vi "BLM Control Text In.vi"(1 "command text in":string[](array[string])=["N/A", "Magent PS", "N/A", "Set Field", "Set Field to 2.0000E+0 @ 0.0000T /min, no wait , extra 0 sec wait", "N/A", "N/A", "", "1", "0", "N/A", "2.000000", "0.000000", "N/A", "N/A", "N/A", "N/A", "N/A", "N/A", "N/A", "N/A", "N/A", "N/A", "N/A", "N/A", "N/A", "N/A", "N/A", "N/A", "N/A", "N/A", "N/A", "N/A", "N/A"]) -> (0 "BLM Control":T1={"extra wait"=0, "Stepper Value"=1e-09, "Value 1"=1.0, "Value 2"=1.0, "String 1"="", "String 2"=""} {"Value 2" format="%#_6e"; "Value 1" format="%<%H:%M:%S>t"; "extra wait" min=0; "Stepper Value" step=0.045 format="%#.7e"})   [LabVIEW 2020]
uses:
  BLM Control.ctl
panel:
  out "Numeric":i32
  # "BLM (Brushless Motor) Control"
  # "(BLM_ManualControl.vi needs to be open before using this program)"
  # "Distance:"
  # "deg of BLM:"
  # "seconds"
  # "AND wait extra"
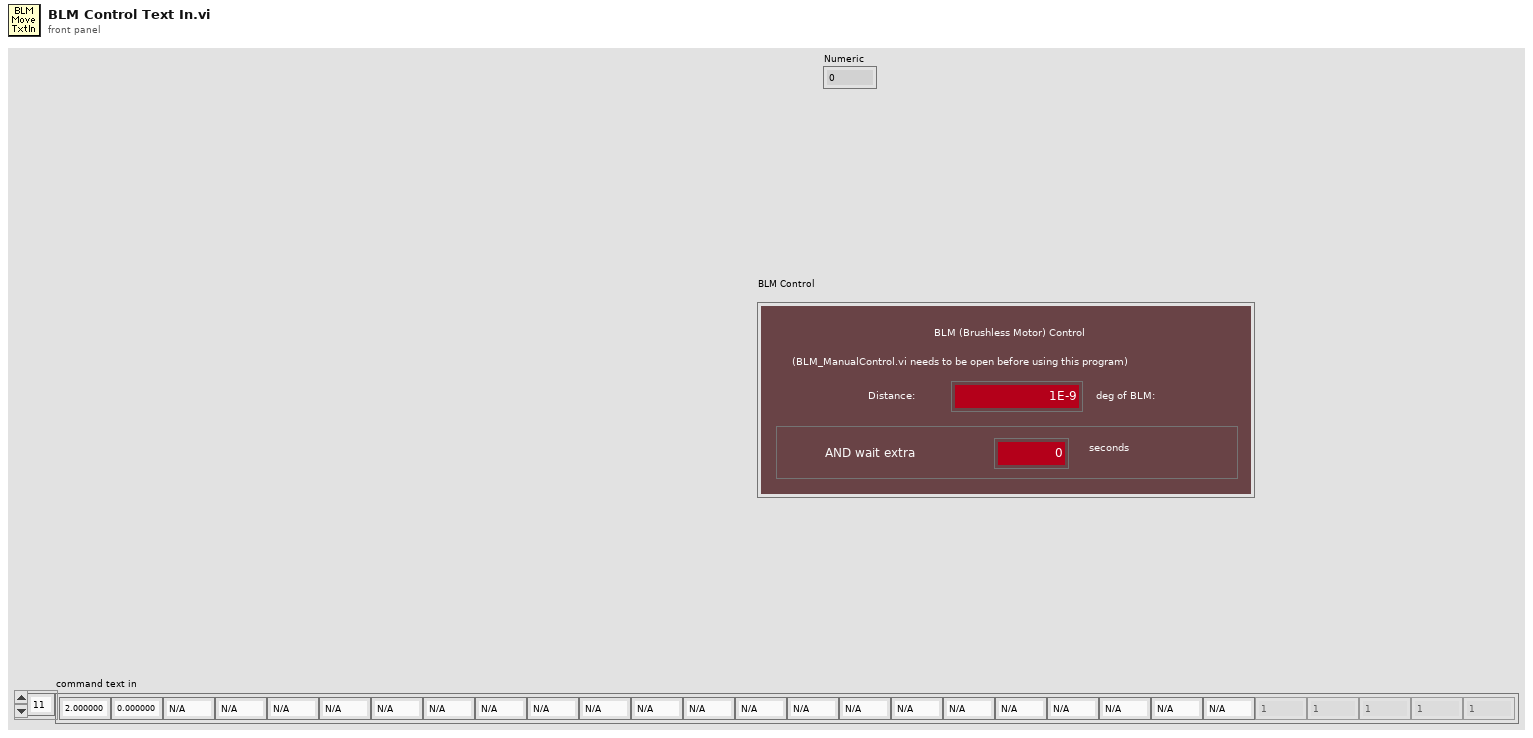
[diagram p1: front panel]
types:
  T1 = typedef "BLM Control.ctl" = cluster{"extra wait":i32, "Stepper Value":dbl, "Value 1":dbl, "Value 2":dbl, "String 1":string, "String 2":string}
  T2 = cluster{"command text in[0]":string, "command text in[1]":string, "command text in[2]":string, "command text in[3]":string, "command text in[4]":string, "command text in[5]":string, "command text in[6]":string, "command text in[7]":string, "command text in[8]":string, "command text in[9]":string, "command text in[10]":string, "command text in[11]":string, "command text in[12]":string, "command text in[13]":string, "command text in[14]":string, "command text in[15]":string, "command text in[16]":string, "command text in[17]":string, "command text in[18]":string, "command text in[19]":string, "command text in[20]":string, "command text in[21]":string, "command text in[22]":string, "command text in[23]":string, "command text in[24]":string, "command text in[25]":string}
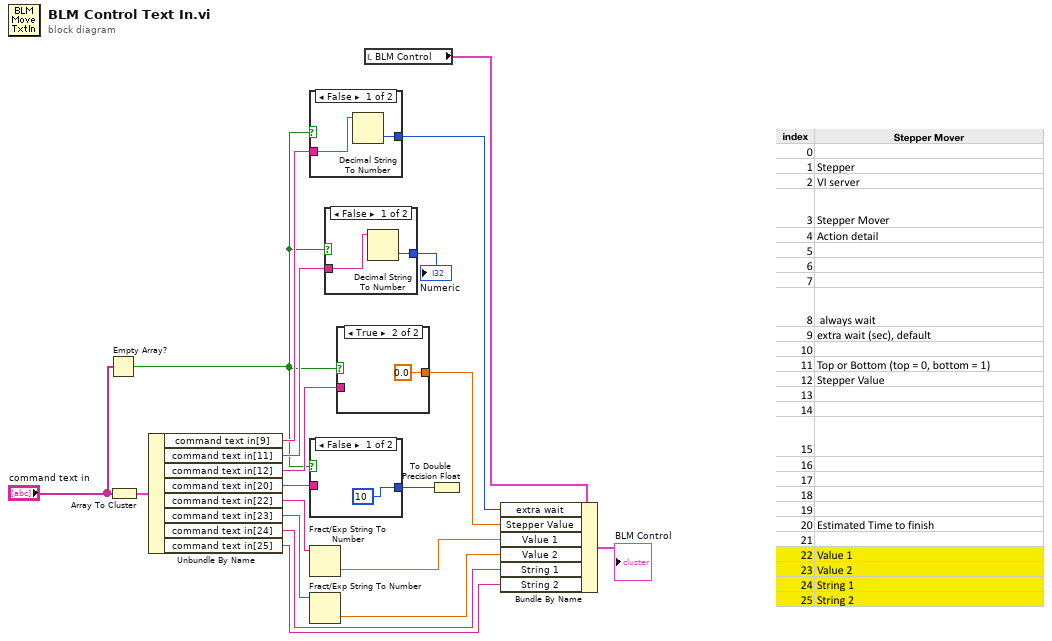
[diagram p0: block diagram]
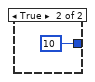
[diagram p2: hidden frame]
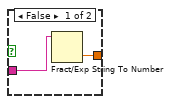
[diagram p3: hidden frame]
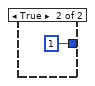
[diagram p4: hidden frame]
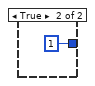
[diagram p5: hidden frame]
diagram:
  n1 = Empty Array?(array="command text in") -> (empty?=w1:bool)
  n2 = Array To Cluster(array="command text in") -> (cluster=w19:T2)
  n3 = Unbundle By Name(w19) -> ("command text in[9]"=w17:string, "command text in[11]"=w16:string, "command text in[12]"=w15:string, "command text in[20]"=w2:string, "command text in[22]"=w10:string, "command text in[23]"=w9:string, "command text in[24]"=w6:string, "command text in[25]"=w5:string)
  n4 = case shown="False" w1 {
    tunnel: w17 -> [w21 _]
    tunnel: [w20 u16 1 ("Value (Signaling)")] -> w12
    frame False {
      n5 = Decimal String To Number(string=w21) -> (number=w20:i32)  [unwired: 2 in, 1 out]
    }
    frame True {
    }
  }
  n6 = case shown="False" w1 {
    tunnel: w2 -> [_ _]
    tunnel: [10 10] -> w3
    frame False {
    }
    frame True {
    }
  }
  n7 = Fract/Exp String To Number(string=w10) -> (number=w8:dbl)  [unwired: 3 in, 1 out]
  n8 = Fract/Exp String To Number(string=w9) -> (number=w7:dbl)  [unwired: 3 in, 1 out]
  n9 = case shown="False" w1 {
    tunnel: w16 -> [w26 _]
    tunnel: [w25 1] -> w11
    frame False {
      n10 = Decimal String To Number(string=w26) -> (number=w25:i32)  [unwired: 2 in, 1 out]
    }
    frame True {
    }
  }
  "Numeric" <- w11
  n11 = case shown="True" w1 {
    tunnel: w15 -> [w28 _]
    tunnel: [w29 0.0] -> w4
    frame False {
      n12 = Fract/Exp String To Number(string=w28) -> (number=w29:dbl)  [unwired: 3 in, 1 out]
    }
    frame True {
    }
  }
  n13 = local read "BLM Control"() -> (w14:T1)
  n14 = To Double Precision Float(number=w3) -> ()  [unwired: 1 out]
  n15 = Bundle By Name(cluster=w14, "extra wait"=w12, "Stepper Value"=w4, "Value 1"=w8, "Value 2"=w7, "String 1"=w6, "String 2"=w5) -> (→"BLM Control":T1)
